vi "main.vi"() -> ()   [LabVIEW 2020]
doc: "This example demonstrates how to acquire a continuous amount of data (Waveform) using the DAQ device's internal clock. It also shows how to synchronize two devices for different device families (E Series, S Series, M Series, X Series, DSA, and SC Express), to simultaneously acquire the data.\n\nFor instructions on how to connect your signals to the DAQ device, refer to your device documentation."
uses:
  <vilib>/Utility/error.llb/DialogType.ctl
  <vilib>/DAQmx/read.llb/DAQmx Read (Analog 1D Wfm NChan NSamp).vi
  <vilib>/DAQmx/configure/timing.llb/DAQmx Timing (Sample Clock).vi
  <vilib>/DAQmx/configure/trigger.llb/DAQmx Start Trigger (Digital Edge).vi
  <vilib>/DAQmx/miscellaneous.llb/DAQmx Fill In Error Info.vi
  <vilib>/Instr/_visa.llb/VISA Configure Serial Port (Instr).vi
panel:
  in  "Pass Logger":T1(tab)=enum."Sense config"
  out "SCD30 CO2 sensor":waveform(dbl)[](graph)=[{"t0"=timestamp(3691127075.8478303 s since 1904-01-01), "dt"=0.0, "Y"=[-35.0]}, {"t0"=timestamp(3691127075.8478303 s since 1904-01-01), "dt"=0.0, "Y"=[0.0]}, {"t0"=timestamp(3691127075.8478303 s since 1904-01-01), "dt"=0.0, "Y"=[0.0]}]
  in  "Stop":bool
  in  "Log":bool=TRUE caption="Enable"
  in  "File config":cluster{"Filepath":path, "Test ID":string}={"Filepath"=path "C:/Users/rhh39/Desktop/NDIR test", "Test ID"="test"}
  out "Lockin - Thermopile voltage":waveform(dbl)[](graph)=[{"t0"=timestamp(3691134575.446129 s since 1904-01-01), "dt"=0.9999799999999999, "Y"=[-1.6384099160002725], "attributes"=variant("NI_ChannelName"=variant(string "Phase - Thermopile Voltage"), "NI_UnitDescription"=variant(string "Rad"))}, {"t0"=timestamp(3691134575.446129 s since 1904-01-01), "dt"=0.9999799999999999, "Y"=[0.1954252740647858], "attributes"=variant("NI_ChannelName"=variant(string "Amplitude - Thermopile Voltage"), "NI_UnitDescription"=variant(string "Volts"))}]
  in  "Sampling":cluster{"Fs":dbl, "#s":dbl}={"Fs"=50000.0, "#s"=50000.0} {"Fs" format="%.2p"}
  out "SCD30":cluster{"CO2":dbl, "Temp (C)":dbl, "RH (%)":dbl}
  in  "CO2 offset":dbl=35.0
  out "Lockin - Heater current":waveform(dbl)[](graph)=[{"t0"=timestamp(3691134575.4461155 s since 1904-01-01), "dt"=0.9999799999999999, "Y"=[-1.004907891175364], "attributes"=variant("NI_ChannelName"=variant(string "Phase - Heater Current"), "NI_UnitDescription"=variant(string "Rad"))}, {"t0"=timestamp(3691134575.4461155 s since 1904-01-01), "dt"=0.9999799999999999, "Y"=[57.2994321062019], "attributes"=variant("NI_ChannelName"=variant(string "Amplitude - Heater Current"), "NI_UnitDescription"=variant(string "mA"))}]
  out "Lockin - Heater voltage":waveform(dbl)[](graph)=[{"t0"=timestamp(3691134575.446122 s since 1904-01-01), "dt"=0.9999799999999999, "Y"=[-1.0832926188523895], "attributes"=variant("NI_ChannelName"=variant(string "Phase - Heater Voltage"), "NI_UnitDescription"=variant(string "Rad"))}, {"t0"=timestamp(3691134575.446122 s since 1904-01-01), "dt"=0.9999799999999999, "Y"=[1.2460360326019546], "attributes"=variant("NI_ChannelName"=variant(string "Amplitude - Heater Voltage"), "NI_UnitDescription"=variant(string "Volts"))}]
  in  "Save waveform":bool=TRUE caption="Enable"
  in  "SCD30":bool caption="Enable"
  out "Lockin output 1":T2={"X"=-0.006601669387256249, "Y"=-0.09748937068791409, "R"=0.0977126370323929, "θ"=-1.6384099160002725, "Amp"=0.1954252740647858, "dt"=0.9999799999999999, "Active channel"="Thermopile Voltage", "Ref channel"="Heater Shunt"} {"X" format="%#_3g"; "Y" format="%#_3g"; "R" format="%#_3g"}
  in  "Config 1":cluster{"Ref Index":i32, "Active Index":i32}={"Ref Index"=0, "Active Index"=2}
  in  "Config 2":cluster{"Ref Index":i32, "Active Index":i32}={"Ref Index"=0, "Active Index"=3}
  out "Lockin output 2":T2={"X"=15.361002717682757, "Y"=-24.183585867911592, "R"=28.64971605310095, "θ"=-1.004907891175364, "Amp"=57.2994321062019, "dt"=0.9999799999999999, "Active channel"="Heater Current", "Ref channel"="Heater Shunt"} {"X" format="%#_3g"; "Y" format="%#_3g"; "R" format="%#_3g"}
  out "Lockin output 3":T2={"X"=0.2918352602557779, "Y"=-0.5504394875979077, "R"=0.6230180163009773, "θ"=-1.0832926188523895, "Amp"=1.2460360326019546, "dt"=0.9999799999999999, "Active channel"="Heater Voltage", "Ref channel"="Heater Shunt"} {"X" format="%#_3g"; "Y" format="%#_3g"; "R" format="%#_3g"}
  in  "Config 3":cluster{"Ref Index":i32, "Active Index":i32}={"Ref Index"=0, "Active Index"=1}
  in  "COM port":refnum<visa-resource-name>="COM16"
  out "AO Waveform Graph":waveform(dbl)(graph)={"t0"=timestamp(0 s since 1904-01-01), "dt"=2e-05, "Y"=array[50000 elements], "attributes"=variant("NI_ChannelName"=variant(string "Heater Mod"), "NI_UnitDescription"=variant(string "Volts"))}
  in  "Channel config":T3={"Frequency"=2.0, "Voltage"=0.9, "Signal type"=enum."Square Wave", "Square wave duty cycle (%)"=50.0, "physical channels"="Dev1/ao0", "name to assign"="Heater Mod", "Phase"=0.0, "Offset"=0.0} {"Square wave duty cycle (%)" format="%0.2f"}
  in  "Config":T4={"Voltage channel index"=1, "Shunt channel index"=0, "Shunt resistance"=10}
  out "Channel names":T5={"Voltage channel name"="Heater Voltage", "Shunt channel name"="Heater Shunt"}
  out "Current Shunt Voltage":waveform(dbl)[](graph)=[{"t0"=timestamp(3691134575.4461155 s since 1904-01-01), "dt"=1.9999999999999998e-05, "Y"=array[50000 elements], "attributes"=variant("NI_ChannelName"=variant(string "Heater Shunt"), "NI_UnitDescription"=variant(string "Volts"))}, {"t0"=timestamp(3691134575.446122 s since 1904-01-01), "dt"=1.9999999999999998e-05, "Y"=array[50000 elements], "attributes"=variant("NI_ChannelName"=variant(string "Heater Voltage"), "NI_UnitDescription"=variant(string "Volts"))}, {"t0"=timestamp(3691134575.446129 s since 1904-01-01), "dt"=1.9999999999999998e-05, "Y"=array[50000 elements], "attributes"=variant("NI_ChannelName"=variant(string "Thermopile Voltage"), "NI_UnitDescription"=variant(string "Volts"))}, {"t0"=timestamp(3691134575.4461155 s since 1904-01-01), "dt"=1.9999999999999998e-05, "Y"=array[50000 elements], "attributes"=variant("NI_ChannelName"=variant(string "Heater Current"), "NI_UnitDescription"=variant(string "mA"))}]
  out "Thermopile Voltage":waveform(dbl)[](graph)=[{"t0"=timestamp(3691134575.4461155 s since 1904-01-01), "dt"=1.9999999999999998e-05, "Y"=array[50000 elements], "attributes"=variant("NI_ChannelName"=variant(string "Heater Shunt"), "NI_UnitDescription"=variant(string "Volts"))}, {"t0"=timestamp(3691134575.446122 s since 1904-01-01), "dt"=1.9999999999999998e-05, "Y"=array[50000 elements], "attributes"=variant("NI_ChannelName"=variant(string "Heater Voltage"), "NI_UnitDescription"=variant(string "Volts"))}, {"t0"=timestamp(3691134575.446129 s since 1904-01-01), "dt"=1.9999999999999998e-05, "Y"=array[50000 elements], "attributes"=variant("NI_ChannelName"=variant(string "Thermopile Voltage"), "NI_UnitDescription"=variant(string "Volts"))}, {"t0"=timestamp(3691134575.4461155 s since 1904-01-01), "dt"=1.9999999999999998e-05, "Y"=array[50000 elements], "attributes"=variant("NI_ChannelName"=variant(string "Heater Current"), "NI_UnitDescription"=variant(string "mA"))}]
  out "Heater Voltage":waveform(dbl)[](graph)=[{"t0"=timestamp(3691134575.4461155 s since 1904-01-01), "dt"=1.9999999999999998e-05, "Y"=array[50000 elements], "attributes"=variant("NI_ChannelName"=variant(string "Heater Shunt"), "NI_UnitDescription"=variant(string "Volts"))}, {"t0"=timestamp(3691134575.446122 s since 1904-01-01), "dt"=1.9999999999999998e-05, "Y"=array[50000 elements], "attributes"=variant("NI_ChannelName"=variant(string "Heater Voltage"), "NI_UnitDescription"=variant(string "Volts"))}, {"t0"=timestamp(3691134575.446129 s since 1904-01-01), "dt"=1.9999999999999998e-05, "Y"=array[50000 elements], "attributes"=variant("NI_ChannelName"=variant(string "Thermopile Voltage"), "NI_UnitDescription"=variant(string "Volts"))}, {"t0"=timestamp(3691134575.4461155 s since 1904-01-01), "dt"=1.9999999999999998e-05, "Y"=array[50000 elements], "attributes"=variant("NI_ChannelName"=variant(string "Heater Current"), "NI_UnitDescription"=variant(string "mA"))}]
  out "Heater Current":waveform(dbl)[](graph)=[{"t0"=timestamp(3691134575.4461155 s since 1904-01-01), "dt"=1.9999999999999998e-05, "Y"=array[50000 elements], "attributes"=variant("NI_ChannelName"=variant(string "Heater Shunt"), "NI_UnitDescription"=variant(string "Volts"))}, {"t0"=timestamp(3691134575.446122 s since 1904-01-01), "dt"=1.9999999999999998e-05, "Y"=array[50000 elements], "attributes"=variant("NI_ChannelName"=variant(string "Heater Voltage"), "NI_UnitDescription"=variant(string "Volts"))}, {"t0"=timestamp(3691134575.446129 s since 1904-01-01), "dt"=1.9999999999999998e-05, "Y"=array[50000 elements], "attributes"=variant("NI_ChannelName"=variant(string "Thermopile Voltage"), "NI_UnitDescription"=variant(string "Volts"))}, {"t0"=timestamp(3691134575.4461155 s since 1904-01-01), "dt"=1.9999999999999998e-05, "Y"=array[50000 elements], "attributes"=variant("NI_ChannelName"=variant(string "Heater Current"), "NI_UnitDescription"=variant(string "mA"))}]
  in  "Channel 2 config":T6={"Channel"="Dev1/ai1", "Vmax"=3.0, "Vmin"=0.0, "name to assign"="Heater Voltage", "input terminal configuration"=10106} {"input terminal configuration" items=["Default"=-1, "RSE"=10083, "NRSE"=10078, "Differential"=10106, "Pseudodifferential"=12529]; "Vmin" format="%0.2f"; "Vmax" format="%0.2f"}
  in  "Channel 1 config":T6={"Channel"="Dev1/ai0", "Vmax"=1.0, "Vmin"=0.0, "name to assign"="Heater Shunt", "input terminal configuration"=10106} {"input terminal configuration" items=["Default"=-1, "RSE"=10083, "NRSE"=10078, "Differential"=10106, "Pseudodifferential"=12529]; "Vmin" format="%0.2f"; "Vmax" format="%0.2f"}
  in  "Channel 3 config":T6={"Channel"="Dev1/ai2", "Vmax"=3.0, "Vmin"=0.0, "name to assign"="Thermopile Voltage", "input terminal configuration"=10106} {"input terminal configuration" items=["Default"=-1, "RSE"=10083, "NRSE"=10078, "Differential"=10106, "Pseudodifferential"=12529]; "Vmin" format="%0.2f"; "Vmax" format="%0.2f"}
  # "PAS Logger"
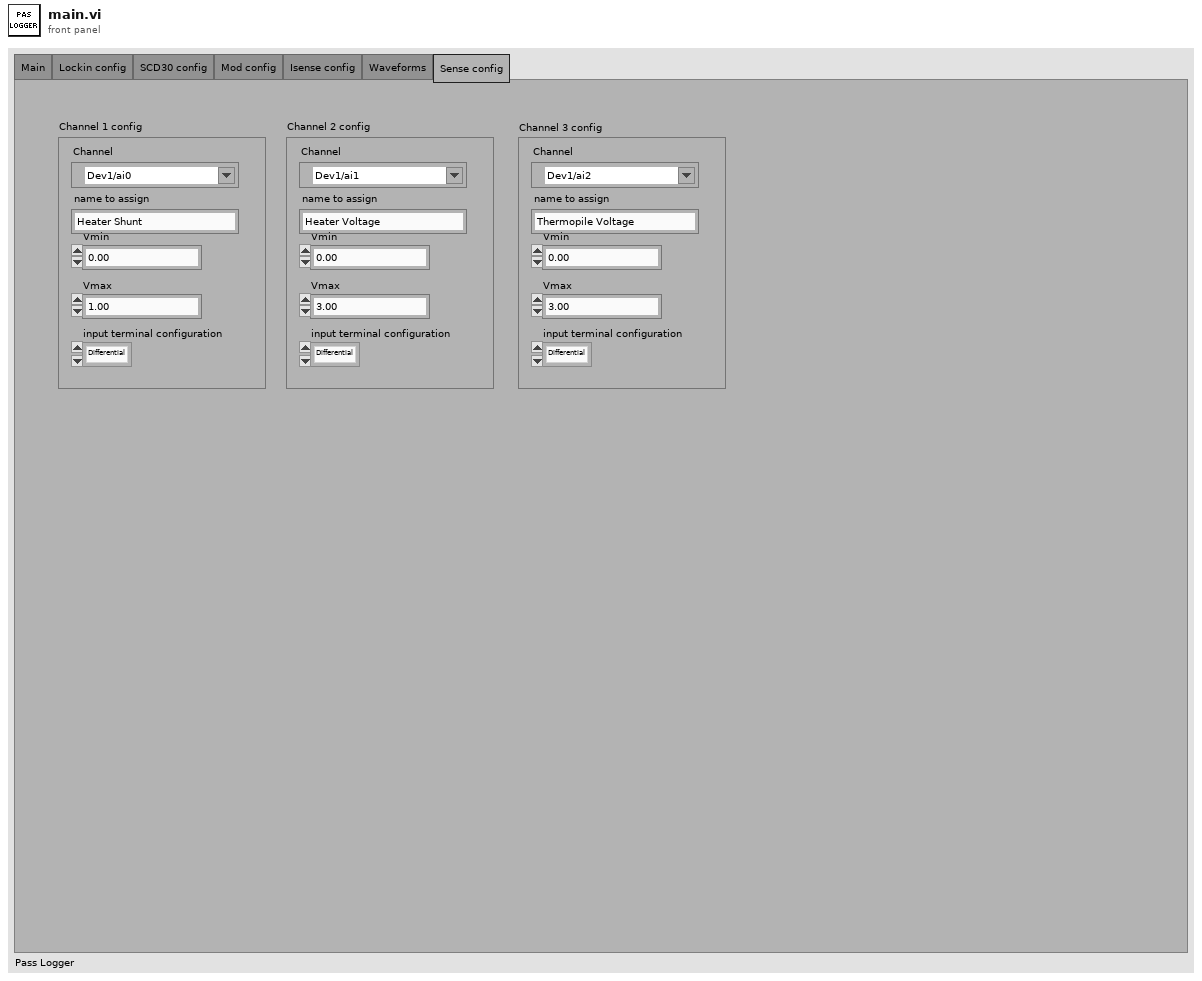
[diagram p1: front panel]
types:
  T1 = enum32{"Main", "Lockin config", "SCD30 config", "Mod config", "Isense config", "Waveforms", "Sense config"}
  T2 = cluster{"X":dbl, "Y":dbl, "R":dbl, "θ":dbl, "Amp":dbl, "dt":dbl, "Active channel":string, "Ref channel":string}
  T3 = cluster{"Frequency":dbl, "Voltage":dbl, "Signal type":enum16{"Sine Wave", "Triangle Wave", "Square Wave", "Sawtooth Wave"}, "Square wave duty cycle (%)":dbl, "physical channels":tag, "name to assign":string, "Phase":dbl, "Offset":dbl}
  T4 = cluster{"Voltage channel index":i32, "Shunt channel index":i32, "Shunt resistance":i32}
  T5 = cluster{"Voltage channel name":string, "Shunt channel name":string}
  T6 = cluster{"Channel":tag, "Vmax":dbl, "Vmin":dbl, "name to assign":string, "input terminal configuration":i32}
  T7 = cluster{"SCD30 CO2":dbl, "SCD30 Temp (C)":dbl, "SCD30 RH (%)":dbl}
  T8 = typedef "DialogType.ctl" = u16
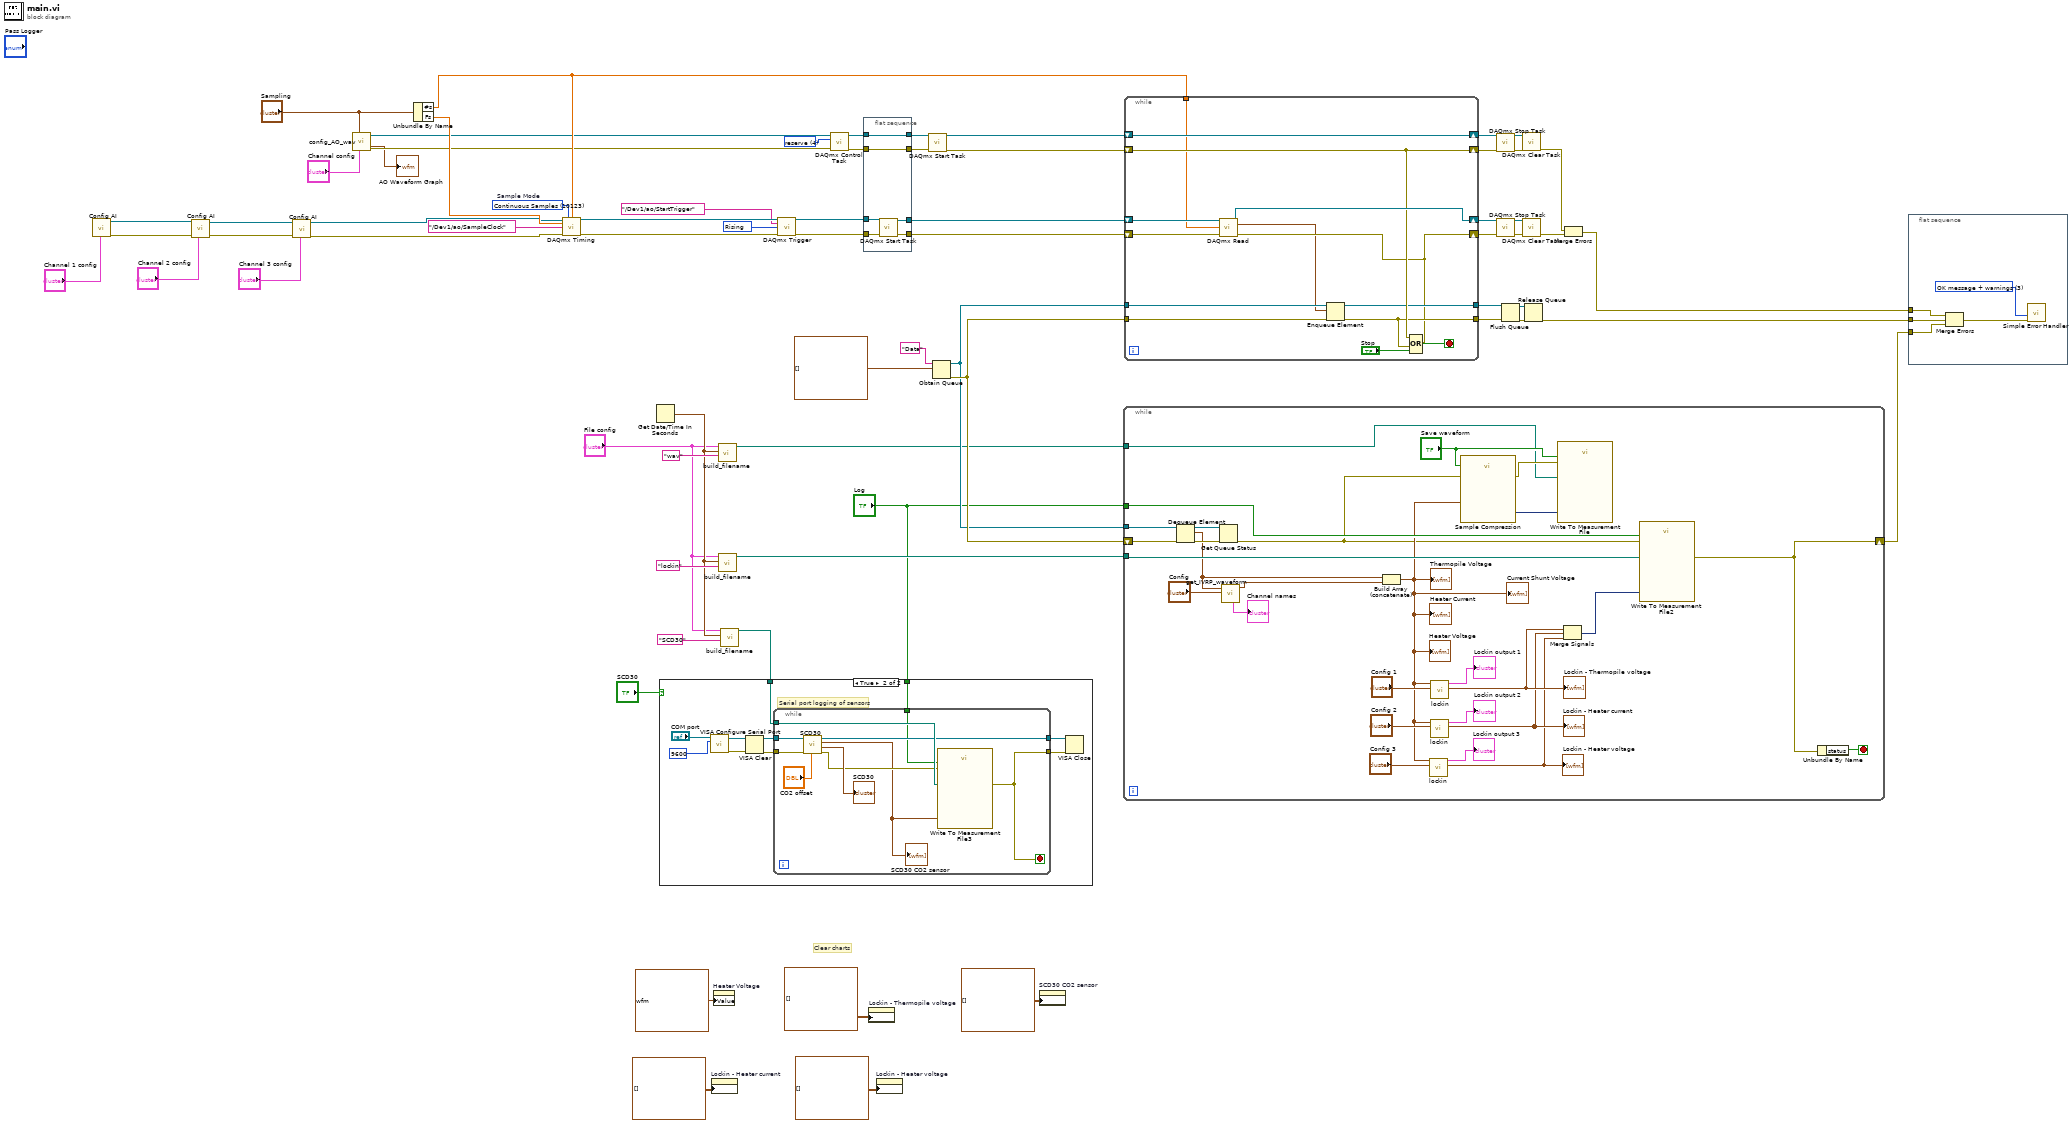
[diagram p0: block diagram]
diagram:
  w51 = 10280 items=["Rising"=10280, "Falling"=10171] ("edge")
  w58 = 4 items=["verify"=2, "reserve"=4, "commit"=3, "unreserve"=5, "abort"=6] ("action")
  w59 = 10123 items=["Finite Samples"=10178, "Continuous Samples"=10123, "Hardware Timed Single Point"=12522]  # Sample Mode
  # "Clear charts"
  n1 = call "Config AI.vi"("Channel config"="Channel 1 config") -> ("error out"=w29:errorcluster, "task out"=w28:refnum<k21>)  [unwired: 9 in]
  n2 = call "Config AI.vi"("Channel config"="Channel 2 config", "error in"=w29, "task in"=w28) -> ("error out"=w14:errorcluster, "task out"=w13:refnum<k21>)  [unwired: 7 in]
  n3 = call "Config AI.vi"("Channel config"="Channel 3 config", "error in"=w14, "task in"=w13) -> ("error out"=w12:errorcluster, "task out"=w11:refnum<k21>)  [unwired: 7 in]
  n4 = call "config_AO_wav.vi"("Channel config"="Channel config", "Sampling info"="Sampling") -> ("error out"=w18:errorcluster, "task out"=w19:refnum<k21>, "AO Waveform Graph"=→"AO Waveform Graph":waveform(dbl))  [unwired: 7 in]
  n5 = Unbundle By Name("Sampling") -> ("#s"=w31:dbl, "Fs"=w30:dbl)
  n6 = call-poly <vilib>:"DAQmx Timing.vi"("task/channels in"=w11, "sample mode"=w59, "samples per channel"=w31, "rate"=w30, "source"=tag "/Dev1/ao/SampleClock", "error in"=w12) -> ("task out"=w52:refnum<k21>, "error out"=w53:errorcluster)  [unwired: 8 in]
  n7 = Get Date/Time In Seconds() -> (seconds since 1Jan1904=w4:timestamp)
  n8 = property on="Lockin - Heater current" class="WFChart (strict)"("History Data"=waveform(dbl)[][] []) -> ()  [unwired: 2 in, 2 out]
  n9 = property on="Heater Voltage" class="WFGraph (strict)"("Value"=waveform(dbl)[] [{"t0"=timestamp(3651561790.263236 s since 1904-01-01), "dt"=0.001, "Y"=array[2000 elements], "attributes"=variant("NI_ChannelName"=variant(string "Mic Active"), "NI_UnitDescription"=variant(string "Volts"))}, {"t0"=timestamp(3651561790.263247 s since 1904-01-01), "dt"=0.001, "Y"=array[2000 elements], "attributes"=variant("NI_ChannelName"=variant(string "Mic Ref"), "NI_UnitDescription"=variant(string "Volts"))}, {"t0"=timestamp(3651561790.263258 s since 1904-01-01), "dt"=0.001, "Y"=array[2000 elements], "attributes"=variant("NI_ChannelName"=variant(string "Diode Heater"), "NI_UnitDescription"=variant(string "Volts"))}, {"t0"=timestamp(3651561790.263269 s since 1904-01-01), "dt"=0.001, "Y"=array[2000 elements], "attributes"=variant("NI_ChannelName"=variant(string "Diode Amb"), "NI_UnitDescription"=variant(string "Volts"))}, {"t0"=timestamp(3651561790.26328 s since 1904-01-01), "dt"=0.001, "Y"=array[2000 elements], "attributes"=variant("NI_ChannelName"=variant(string "Heater Shunt"), "NI_UnitDescription"=variant(string "Volts"))}, {"t0"=timestamp(3651561790.2632914 s since 1904-01-01), "dt"=0.001, "Y"=array[2000 elements], "attributes"=variant("NI_ChannelName"=variant(string "Heater V"), "NI_UnitDescription"=variant(string "Volts"))}, {"t0"=timestamp(3651561790.263247 s since 1904-01-01), "dt"=0.001, "Y"=array[2000 elements], "attributes"=variant("NI_ChannelName"=variant(string "Mic Diff"), "NI_UnitDescription"=variant(string "Volts"))}, {"t0"=timestamp(3651561790.26328 s since 1904-01-01), "dt"=0.001, "Y"=array[2000 elements], "attributes"=variant("NI_ChannelName"=variant(string "Heater Current"), "NI_UnitDescription"=variant(string "Amps"))}] ("Waveform")) -> ()  [unwired: 2 in, 2 out]
  n10 = call "build_filename.vi"("Test type"="wav" ("File Descriptor"), "time stamp"=w4, "File config"="File config") -> ("appended path"=w3:path)  [unwired: 8 in]
  n11 = call "build_filename.vi"("Test type"="lockin" ("File Descriptor"), "time stamp"=w4, "File config"="File config") -> ("appended path"=w24:path)  [unwired: 8 in]
  n12 = call "build_filename.vi"("Test type"="SCD30" ("File Descriptor"), "time stamp"=w4, "File config"="File config") -> ("appended path"=w7:path)  [unwired: 8 in]
  n13 = case shown="True" "SCD30" {
    tunnel: w7 -> [_ w71]
    tunnel: "Log" -> [_ w70]
    frame False {
    }
    frame True {
      # "Serial port logging of sensors"
      n14 = call-poly "VISA Configure Serial Port"("VISA resource name"="COM port", "baud rate (9600)"=u32 9600) -> ("VISA resource name out"=w75:refnum<visa-resource-name>, "error out"=w74:errorcluster)  [unwired: 7 in, 5 out]
      n15 = VISA Clear(VISA resource name=w75, error in (no error)=w74) -> (VISA resource name out=w76:refnum<visa-resource-name>, error out=w77:errorcluster)
      n16 = while {
        tunnel: w76 -> [w87]
        tunnel: w77 -> [w86]
        tunnel: [w88] -> w78
        tunnel: [w82] -> w79
        tunnel: w71 -> [w89]
        tunnel: w70 -> [w80]
        stop <- w88 stop-if-true
        n17 = call "SCD30.vi"("CO2 offset"="CO2 offset", "error in (no error)"=w86, "VISA resource name"=w87) -> ("error out"=w84:errorcluster, "Readings"=→"SCD30":T7, "appended array"=w83:waveform(dbl)[], "VISA resource name out"=w82:refnum<visa-resource-name>)  [unwired: 5 in]
        "SCD30 CO2 sensor" <- w83
        n18 = call "Write To Measurement File3"("Signals"=w83, "Enable"=w80, "error in (no error)"=w84, "Filename"=w89) -> ("error out"=w88:errorcluster)  [unwired: 13 in, 2 out]
      }
      n19 = VISA Close(VISA resource name=w79, error in (no error)=w78) -> ()  [unwired: 1 out]
    }
  }
  n20 = call-poly <vilib>:"DAQmx Trigger.vi"("task/channels in"=w52, "source"=tag "/Dev1/ao/StartTrigger", "edge"=w51, "error in"=w53) -> ("task out"=w49:refnum<k21>, "error out"=w50:errorcluster)  [unwired: 10 in]
  n21 = call <vilib>:"DAQmx Control Task.vi"("task/channels in"=w19, "action"=w58, "error in"=w18) -> ("task out"=w48:refnum<k21>, "error out"=w46:errorcluster)  [unwired: 11 in]
  n22 = flat-sequence {
    tunnel: [w95] -> w55
    tunnel: [w94] -> w54
    tunnel: w50 -> [w93]
    tunnel: w49 -> [w92]
    tunnel: w48 -> [w91]
    tunnel: [w91] -> w47
    tunnel: w46 -> [w90]
    tunnel: [w90] -> w45
    frame #0 {
      n23 = call <vilib>:"DAQmx Start Task.vi"("task/channels in"=w92, "error in"=w93) -> ("task out"=w94:refnum<k21>, "error out"=w95:errorcluster)  [unwired: 12 in]
    }
  }
  n24 = property on="Lockin - Thermopile voltage" class="WFChart (strict)"("History Data"=waveform(dbl)[][] []) -> ()  [unwired: 2 in, 2 out]
  n25 = property on="Lockin - Heater voltage" class="WFChart (strict)"("History Data"=waveform(dbl)[][] []) -> ()  [unwired: 2 in, 2 out]
  n26 = call <vilib>:"DAQmx Start Task.vi"("task/channels in"=w47, "error in"=w45) -> ("task out"=w56:refnum<k21>, "error out"=w57:errorcluster)  [unwired: 12 in]
  n27 = Obtain Queue(name (unnamed)="Data" ("名前（名前なし）"), element data type=waveform(dbl)[] [] ("data")) -> (queue out=w34:refnum<queue>, error out=w35:errorcluster)  [unwired: 3 in, 1 out]
  n28 = property on="SCD30 CO2 sensor" class="WFChart (strict)"("History Data"=waveform(dbl)[][] []) -> ()  [unwired: 2 in, 2 out]
  n29 = while {
    tunnel: w34 -> [w122]
    shift-right: [w102] -> w33
    shift-left: w35 -> [w123]
    tunnel: w24 -> [w119]
    tunnel: "Log" -> [w111]
    tunnel: w3 -> [w96]
    stop <- w118 stop-if-true
    n30 = Dequeue Element(queue=w122, error in (no error)=w123) -> (queue out=w120:refnum<queue>, element=w112:waveform(dbl)[], error out=w121:errorcluster)  [unwired: 1 in, 1 out]
    n31 = Get Queue Status(queue=w120, error in (no error)=w121) -> (error out=w99:errorcluster)  [unwired: 1 in, 7 out]
    n32 = call "get_IVRP_waveform.vi"("Channel config"="Config", "array"=w112) -> ("Current waveform out"=w113:waveform(dbl), "Channel names"=→"Channel names":T5)  [unwired: 5 in, 3 out]
    n33 = Build Array (concatenate)(w112, w113) -> (w101:waveform(dbl)[])
    "Heater Voltage" <- w101
    "Heater Current" <- w101
    "Thermopile Voltage" <- w101
    "Current Shunt Voltage" <- w101
    n34 = call "lockin.vi"("Config"="Config 3", "array"=w101) -> ("Output waveform"=w104:waveform(dbl)[], "Lockin output"=→"Lockin output 3":T2)  [unwired: 8 in]
    "Lockin - Heater voltage" <- w104
    n35 = call "lockin.vi"("Config"="Config 2", "array"=w101) -> ("Output waveform"=w105:waveform(dbl)[], "Lockin output"=→"Lockin output 2":T2)  [unwired: 8 in]
    "Lockin - Heater current" <- w105
    n36 = call "lockin.vi"("Config"="Config 1", "array"=w101) -> ("Output waveform"=w106:waveform(dbl)[], "Lockin output"=→"Lockin output 1":T2)  [unwired: 8 in]
    "Lockin - Thermopile voltage" <- w106
    n37 = call "Sample Compression"("error in (no error)"=w99, "Enable"="Save waveform", "Signals"=w101) -> ("error out"=w98:errorcluster, "Mean"=w100:dynamicdata)  [unwired: 6 in, 1 out]
    n38 = call "Write To Measurement File"("Signals"=w100, "Enable"="Save waveform", "error in (no error)"=w98, "Filename"=w96) -> ()  [unwired: 13 in, 3 out]
    n39 = Merge Signals(w106, w105, w104) -> (w103:dynamicdata)
    n40 = call "Write To Measurement File2"("Signals"=w103, "Enable"=w111, "error in (no error)"=w99, "Filename"=w119) -> ("error out"=w102:errorcluster)  [unwired: 13 in, 2 out]
    n41 = Unbundle By Name(w102) -> ("status"=w118:bool)
  }
  n42 = while {
    shift-right: [w133] -> w68
    shift-left: w57 -> [w133]
    shift-right: [w125] -> w64
    shift-left: w55 -> [w135]
    shift-right: [w132] -> w69
    shift-left: w56 -> [w132]
    shift-right: [w134] -> w65
    shift-left: w54 -> [w136]
    tunnel: w31 -> [w131]
    tunnel: [w130] -> w40
    tunnel: [w126] -> w39
    tunnel: w34 -> [w129]
    tunnel: w35 -> [w128]
    stop <- w137 stop-if-true
    n43 = call-poly <vilib>:"DAQmx Read.vi"("task/channels in"=w136, "number of samples per channel"=w131, "error in"=w135) -> ("task out"=w134:refnum<k21>, "data"=w124:waveform(dbl)[], "error out"=w125:errorcluster)  [unwired: 10 in]
    n44 = Enqueue Element(queue=w129, element=w124, error in (no error)=w128) -> (queue out=w130:refnum<queue>, error out=w126:errorcluster)  [unwired: 1 in, 1 out]
    n45 = Compound Arithmetic op=OR(w133, w125, w126, "Stop") -> (w137:bool)
  }
  n46 = call <vilib>:"DAQmx Stop Task.vi"("task/channels in"=w69, "error in"=w68) -> ("task out"=w66:refnum<k21>, "error out"=w67:errorcluster)  [unwired: 12 in]
  n47 = call <vilib>:"DAQmx Stop Task.vi"("task/channels in"=w65, "error in"=w64) -> ("task out"=w62:refnum<k21>, "error out"=w63:errorcluster)  [unwired: 12 in]
  n48 = Flush Queue(queue=w40, error in (no error)=w39) -> (queue out=w41:refnum<queue>, error out=w42:errorcluster)  [unwired: 1 out]
  n49 = call <vilib>:"DAQmx Clear Task.vi"("task in"=w66, "error in"=w67) -> ("error out"=w61:errorcluster)  [unwired: 13 in]
  n50 = call <vilib>:"DAQmx Clear Task.vi"("task in"=w62, "error in"=w63) -> ("error out"=w60:errorcluster)  [unwired: 13 in]
  n51 = Release Queue(queue=w41, error in (no error)=w42) -> (error out=w37:errorcluster)  [unwired: 1 in, 2 out]
  n52 = Merge Errors(w61, w60) -> (w38:errorcluster)
  n53 = flat-sequence {
    tunnel: w38 -> [w142]
    tunnel: w37 -> [w141]
    tunnel: w33 -> [w138]
    frame #0 {
      w140 = T8 3 items=["no dialog", "OK message", "continue or stop message", "OK message + warnings", "continue/stop + warnings"] ("type of dialog (OK msg:1)")
      n54 = Merge Errors(w142, w141, w138) -> (w139:errorcluster)
      n55 = call <vilib>:"Simple Error Handler.vi"("type of dialog (OK msg:1)"=w140, "error in (no error)"=w139) -> ()  [unwired: 3 in, 5 out]
    }
  }
